vi "Set Auto-Scroll.vi"(8 "error in (no error)":errorcluster, 10 "Auto-Scroll?":bool, 11 "Chronological List in":refnum<class "Chronological List.lvclass">) -> (0 "error out":errorcluster, 3 "Chronological List out":refnum<class "Chronological List.lvclass">)   [LabVIEW 2020, in "Chronological List.lvclass"]
uses:
  Chronological List.lvclass
  Chronological List.lvclass/Chronological List.ctl
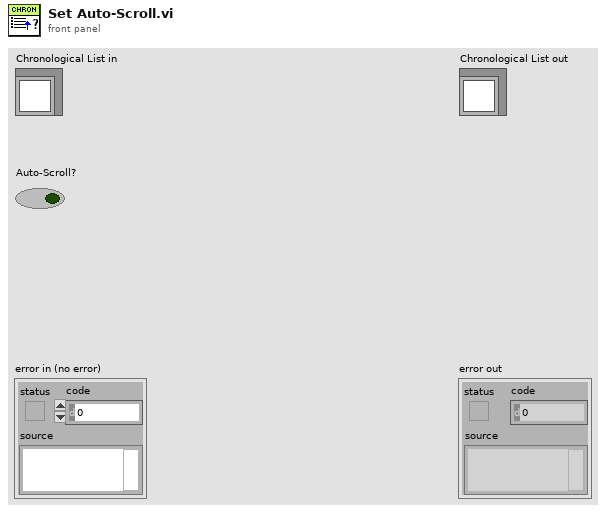
[diagram p1: front panel]
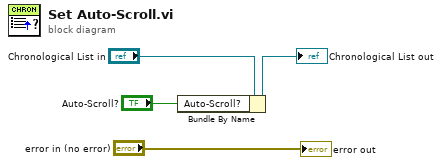
[diagram p0: block diagram]
diagram:
  n1 = Bundle By Name(cluster="Chronological List in", "Auto-Scroll?"="Auto-Scroll?") -> (→"Chronological List out":refnum<class "Chronological List.lvclass">)
  "error out" <- "error in (no error)"
